vi "Get Project Ref and Name.vi"(11 "Project Name Selection":string) -> (3 "Project":T1)   [LabVIEW 2020, in "Panther Dashboard.lvlib"]
uses:
  Panther Dashboard.lvlib
  Project Name and Ref--cluster.ctl
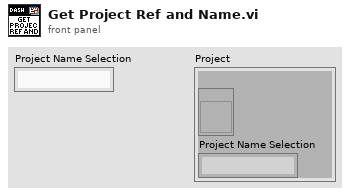
[diagram p1: front panel]
types:
  T1 = typedef "Panther Dashboard.lvlib/Project Name and Ref--cluster.ctl" = cluster{"Project Ref":refnum<vi>, "Project Name Selection":string}
  T2 = cluster{refnum<vi>, "Project Name Selection":string}
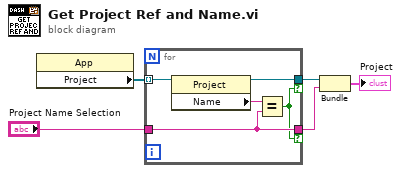
[diagram p0: block diagram]
diagram:
  n1 = property class="App"() -> ("Project"=w4:refnum<vi>[])  [unwired: 2 in, 2 out]
  n2 = for {
    tunnel: w4 -> [w10] mode=indexing
    tunnel: "Project Name Selection" -> [w7]
    tunnel: [w9] -> w3 if=w6
    tunnel: [w7] -> w2 if=w6
    n3 = property class="Project"(reference=w10) -> (reference out=w9:refnum<vi>, "Name"=w8:string)  [unwired: 1 in, 1 out]
    n4 = Equal?(x=w8, y=w7) -> (x = y?=w6:bool)
  }
  n5 = Bundle(w3, "Project Name Selection"=w2) -> (→"Project":T2)  [unwired: 1 in]
